vi "NR Configure Standard.vi"(0 "RFmx Handle In":refnum<k21>, 1 "Selector String":string, 5 "NR Standard Configuration":T1={"Link Direction"=1, "Frequency Range"=0, "Band"=78, "Auto Resource Block Detection Enabled"=1, "Downlink Test Model"=0, "Downlink Test Model Duplex Scheme"=0, "Component Carrier Configurations"=[{"Bandwidth (Hz)"=100000000.0, "Cell ID"=0, "PUSCH Modulation Type"=1, "Subcarrier Spacing (Hz)"=30000.0, "PUSCH Resource Block Offset"=0, "PUSCH Number of Resource Blocks"=-1, "PUSCH Transform Precoding Enabled"=0, "PUSCH Slot Allocation"="0-Last", "PUSCH Symbol Allocation"="0-Last", "PUSCH DMRS Configuration Type"=0, "PUSCH Mapping Type"=0, "PUSCH DMRS Type A Position"=2, "PUSCH DMRS Duration"=1, "PUSCH DMRS Additional Positions"=0}]} {"Downlink Test Model Duplex Scheme" items=["FDD", "TDD"]; "Downlink Test Model" items=["TM1.1", "TM1.2", "TM2", "TM2a", "TM3.1", "TM3.1a", "TM3.2", "TM3.3"]; "Component Carrier Configurations"."PUSCH DMRS Additional Positions" items=["0", "1", "2", "3"]; "Component Carrier Configurations"."PUSCH DMRS Duration" items=["Single-Symbol"=1, "Double-Symbol"=2]; "Component Carrier Configurations"."PUSCH DMRS Type A Position" items=["2"=2, "3"=3]; "Component Carrier Configurations"."PUSCH Mapping Type" items=["Type A", "Type B"]; "Component Carrier Configurations"."PUSCH DMRS Configuration Type" items=["Type 1", "Type 2"]; "Component Carrier Configurations"."PUSCH Transform Precoding Enabled" items=["False", "True"]; "Component Carrier Configurations"."Subcarrier Spacing (Hz)" items=["15kHz"=15000.0, "30kHz"=30000.0, "60kHz"=60000.0, "120kHz"=120000.0]; "Component Carrier Configurations"."PUSCH Modulation Type" items=["PI/2 BPSK", "QPSK", "16 QAM", "64 QAM", "256 QAM"]; "Component Carrier Configurations"."Bandwidth (Hz)" items=["5M"=5000000.0, "10M"=10000000.0, "15M"=15000000.0, "20M"=20000000.0, "25M"=25000000.0, "30M"=30000000.0, "40M"=40000000.0, "50M"=50000000.0, "60M"=60000000.0, "70M"=70000000.0, "80M"=80000000.0, "90M"=90000000.0, "100M"=100000000.0, "200M"=200000000.0, "400M"=400000000.0]; "Auto Resource Block Detection Enabled" items=["False", "True"]; "Frequency Range" items=["Range 1", "Range 2"]; "Link Direction" items=["Downlink", "Uplink"]}, 11 "error in (no error)":errorcluster) -> (4 "RFmx Handle Out":refnum<k21>, 15 "error out":errorcluster)   [LabVIEW 2016, in "RFmxNR.lvlib"]
uses:
  RFmxNR.lvlib
  Typedefs/NR Standard Configuration.ctl
  <resource>/objmgr/RFmxNR.rc
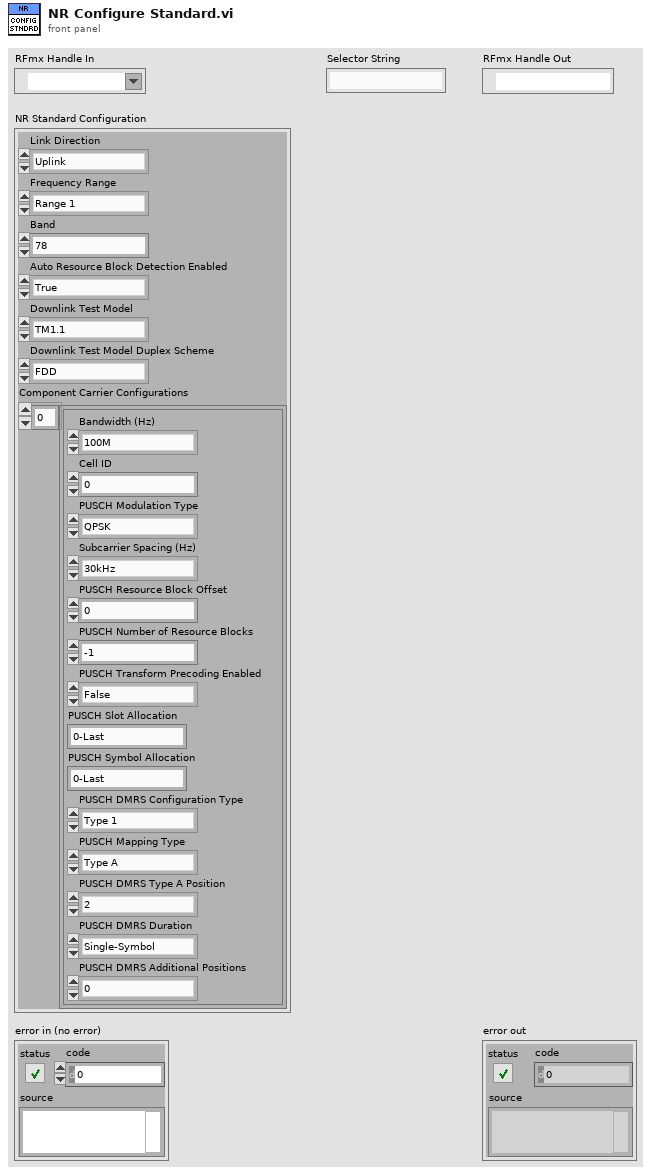
[diagram p1: front panel]
types:
  T1 = typedef "RFmxNR.lvlib/NR Standard Configuration.ctl" = cluster{"Link Direction":i32, "Frequency Range":i32, "Band":i32, "Auto Resource Block Detection Enabled":i32, "Downlink Test Model":i32, "Downlink Test Model Duplex Scheme":i32, "Component Carrier Configurations":cluster{"Bandwidth (Hz)":dbl, "Cell ID":i32, "PUSCH Modulation Type":i32, "Subcarrier Spacing (Hz)":dbl, "PUSCH Resource Block Offset":i32, "PUSCH Number of Resource Blocks":i32, "PUSCH Transform Precoding Enabled":i32, "PUSCH Slot Allocation":string, "PUSCH Symbol Allocation":string, "PUSCH DMRS Configuration Type":i32, "PUSCH Mapping Type":i32, "PUSCH DMRS Type A Position":i32, "PUSCH DMRS Duration":i32, "PUSCH DMRS Additional Positions":i32}[]}
  T2 = cluster{"Bandwidth (Hz)":dbl, "Cell ID":i32, "PUSCH Modulation Type":i32, "Subcarrier Spacing (Hz)":dbl, "PUSCH Resource Block Offset":i32, "PUSCH Number of Resource Blocks":i32, "PUSCH Transform Precoding Enabled":i32, "PUSCH Slot Allocation":string, "PUSCH Symbol Allocation":string, "PUSCH DMRS Configuration Type":i32, "PUSCH Mapping Type":i32, "PUSCH DMRS Type A Position":i32, "PUSCH DMRS Duration":i32, "PUSCH DMRS Additional Positions":i32}[]
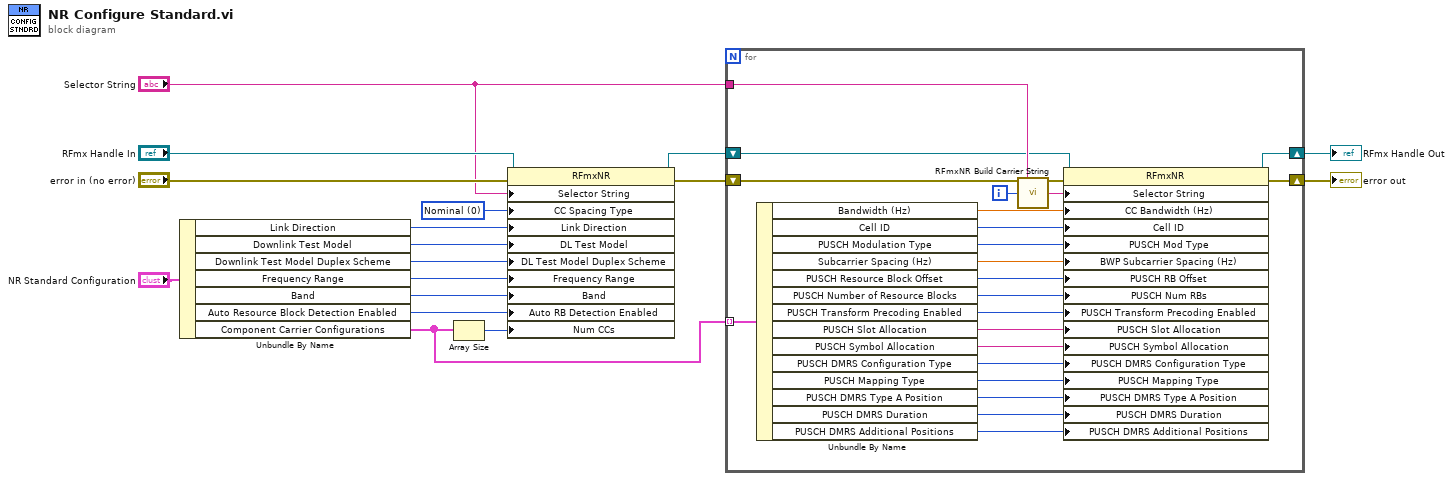
[diagram p0: block diagram]
diagram:
  w17 = 0 items=["Nominal"=0, "User"=2] ("CC Spacing Type")
  n1 = Unbundle By Name("NR Standard Configuration") -> ("Link Direction"=w14:i32, "Downlink Test Model"=w2:i32, "Downlink Test Model Duplex Scheme"=w1:i32, "Frequency Range"=w13:i32, "Band"=w12:i32, "Auto Resource Block Detection Enabled"=w11:i32, "Component Carrier Configurations"=w3:T2)
  n2 = Array Size(array=w3) -> (size(s)=w10:i32)
  n3 = property class="RFmxNR"(reference="RFmx Handle In", error in="error in (no error)", "Selector String"="Selector String", "CC Spacing Type"=w17, "Link Direction"=w14, "DL Test Model"=w2, "DL Test Model Duplex Scheme"=w1, "Frequency Range"=w13, "Band"=w12, "Auto RB Detection Enabled"=w11, "Num CCs"=w10) -> (reference out=w6:refnum<k21>, error out=w7:errorcluster)
  n4 = for {
    shift-right: [w34] -> w8
    shift-left: w7 -> [w37]
    shift-right: [w35] -> w5
    shift-left: w6 -> [w36]
    tunnel: w3 -> [w33] mode=indexing
    tunnel: "Selector String" -> [w39]
    i -> [w38]
    n5 = Unbundle By Name(w33) -> ("Bandwidth (Hz)"=w32:dbl, "Cell ID"=w31:i32, "PUSCH Modulation Type"=w30:i32, "Subcarrier Spacing (Hz)"=w29:dbl, "PUSCH Resource Block Offset"=w28:i32, "PUSCH Number of Resource Blocks"=w27:i32, "PUSCH Transform Precoding Enabled"=w26:i32, "PUSCH Slot Allocation"=w25:string, "PUSCH Symbol Allocation"=w24:string, "PUSCH DMRS Configuration Type"=w23:i32, "PUSCH Mapping Type"=w22:i32, "PUSCH DMRS Type A Position"=w21:i32, "PUSCH DMRS Duration"=w20:i32, "PUSCH DMRS Additional Positions"=w19:i32)
    n6 = call <vilib>:"RFmxNR Build Carrier String.vi"("Selector String"=w39, "Carrier Number"=w38) -> ("Selector String Out"=w18:string)  [unwired: 13 in]
    n7 = property class="RFmxNR"(reference=w36, error in=w37, "Selector String"=w18, "CC Bandwidth (Hz)"=w32, "Cell ID"=w31, "PUSCH Mod Type"=w30, "BWP Subcarrier Spacing (Hz)"=w29, "PUSCH RB Offset"=w28, "PUSCH Num RBs"=w27, "PUSCH Transform Precoding Enabled"=w26, "PUSCH Slot Allocation"=w25, "PUSCH Symbol Allocation"=w24, "PUSCH DMRS Configuration Type"=w23, "PUSCH Mapping Type"=w22, "PUSCH DMRS Type A Position"=w21, "PUSCH DMRS Duration"=w20, "PUSCH DMRS Additional Positions"=w19) -> (reference out=w35:refnum<k21>, error out=w34:errorcluster)
  }
  "error out" <- w8
  "RFmx Handle Out" <- w5
